vi "Launcher.vi"() -> ()   [LabVIEW 2019]
uses:
  <vilib>/ActorFramework/Message Enqueuer/Message Enqueuer.lvclass
  Status Actor/Status Actor.lvclass
  C:/Program Files/National Instruments/LabVIEW 2019/vi.lib/ActorFramework/Actor/Actor.lvclass
  Generador de funciones/Generador de funciones.lvclass
  <vilib>/ActorFramework/Message Enqueuer/Message Enqueuer.lvclass/Message Enqueuer.ctl
  <vilib>/ActorFramework/Message Enqueuer/Enqueue.vi
  <vilib>/ActorFramework/Stop Msg/Stop Msg.lvclass
  C:/Program Files/National Instruments/LabVIEW 2019/vi.lib/ActorFramework/Message/Message.lvclass
  <vilib>/ActorFramework/Message Priority Queue/Priority Enqueue.vi
  <vilib>/ActorFramework/Actor/Actor.lvclass
panel:
  in  "Exit":bool
  in  "Active Actors":u16(ring) items=["", "1"]
  in  "Stop Selected Actor":bool
  in  "Tipo de Actor":u16(ring) items=["Select an actor", "Status Actor", "Generador Actor"]
  in  "New Actor":bool
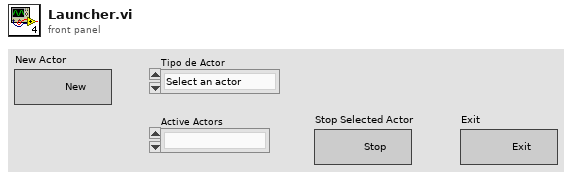
[diagram p1: front panel]
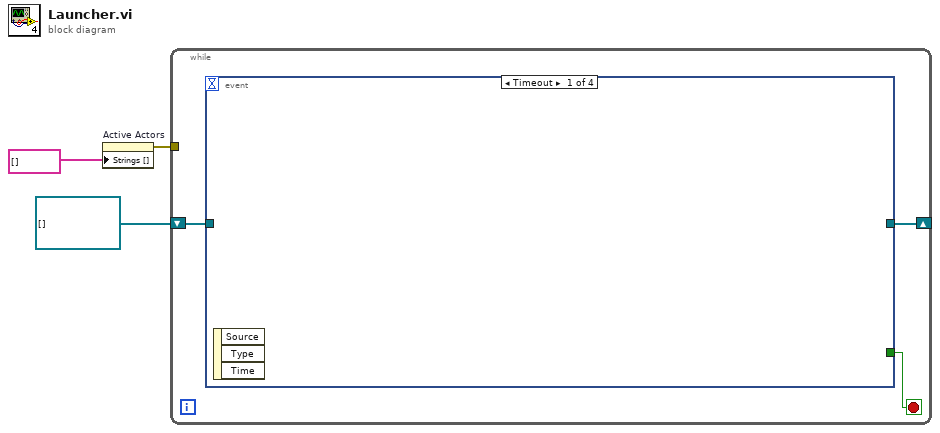
[diagram p0: block diagram]
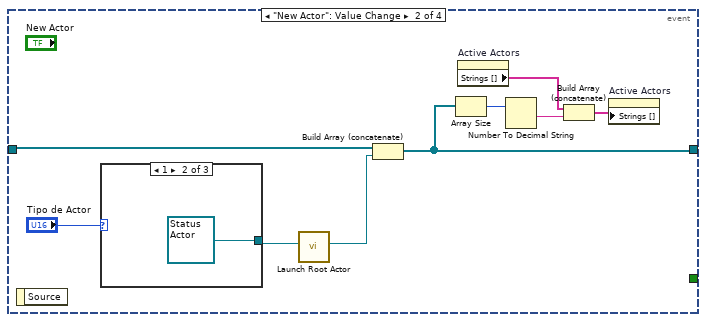
[diagram p2: hidden frame]
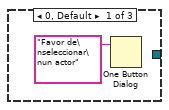
[diagram p3: hidden frame]
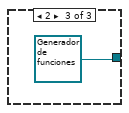
[diagram p4: hidden frame]
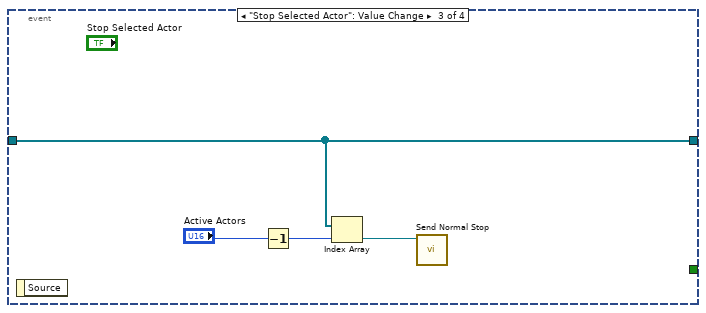
[diagram p5: hidden frame]
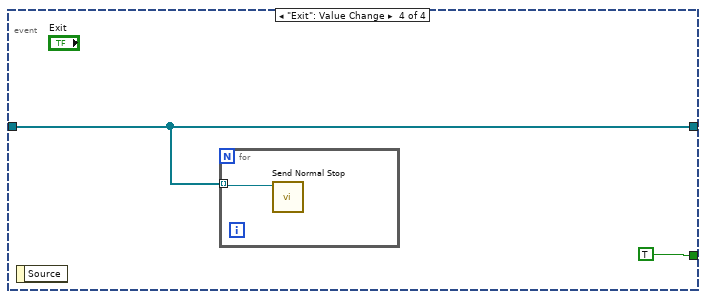
[diagram p6: hidden frame]
diagram:
  n1 = property on="Active Actors" class="Ring (strict)"("Strings []"=string[] []) -> (error out=w1:errorcluster)  [unwired: 2 in, 1 out]
  n2 = while {
    shift-right: [w5] -> _
    shift-left: refnum<class "Message Enqueuer.lvclass">[] [] ("Array") -> [w6]
    tunnel: w1 -> [_]
    stop <- w4 stop-if-true
    n3 = event shown="[0] Timeout" {
      selector: _ -> [_ _ _ _]
      dyn-events: _ -> [_ _ _ _]
      timeout: _ -> [_ _ _ _]
      tunnel: w6 -> [_ w12 w20 w23]
      tunnel: [_ w10 w20 w23] -> w5
      tunnel: [_ _ _ TRUE] -> w4
      event Timeout {
        n4 = event-data() -> ()  [unwired: 1 in, 3 out]
      }
      event "New Actor": Value Change {
        n5 = event-data() -> ()  [unwired: 1 in, 1 out]
        n6 = case shown="1" "Tipo de Actor" {
          tunnel: [_ refnum<class "Status Actor.lvclass"> refnum ("Status Actor.lvlib:Status Actor.lvclass") refnum<class "Generador de funciones.lvclass"> refnum ("Generador de funciones.lvlib:Generador de funciones.lvclass")] -> w13
          frame 0, Default {
            n7 = One Button Dialog(message="Favor de\nseleccionar\nun actor") -> ()  [unwired: 1 in, 1 out]
          }
          frame 1 {
          }
          frame 2 {
          }
        }
        n8 = call <vilib>:"Launch Root Actor.vi"("Actor"=w13) -> ("Actor's Enqueuer"=w11:refnum<class "Message Enqueuer.lvclass">)  [unwired: 9 in, 1 out]
        n9 = Build Array (concatenate)(w12, w11) -> (w10:refnum<class "Message Enqueuer.lvclass">[])
        n10 = Array Size(array=w10) -> (size(s)=w15:i32)
        n11 = property on="Active Actors" class="Ring (strict)"() -> ("Strings []"=w9:string[])  [unwired: 2 in, 2 out]
        n12 = Number To Decimal String(number=w15) -> (decimal integer string=w14:string)  [unwired: 1 in]
        n13 = Build Array (concatenate)(w9, w14) -> (w8:string[])
        n14 = property on="Active Actors" class="Ring (strict)"("Strings []"=w8) -> ()  [unwired: 2 in, 2 out]
      }
      event "Stop Selected Actor": Value Change {
        n15 = event-data() -> ()  [unwired: 1 in, 1 out]
        n16 = Decrement(x="Active Actors") -> (x-1=w22:u16)
        n17 = Index Array "Index Array"(array=w20, index=w22) -> (element=w19:refnum<class "Message Enqueuer.lvclass">)
        n18 = call <vilib>:"Send Normal Stop.vi"("Message Enqueuer"=w19) -> ()  [unwired: 10 in, 1 out]
      }
      event "Exit": Value Change {
        n19 = event-data() -> ()  [unwired: 1 in, 1 out]
        n20 = for {
          tunnel: w23 -> [w25] mode=indexing
          n21 = call <vilib>:"Send Normal Stop.vi"("Message Enqueuer"=w25) -> ()  [unwired: 10 in, 1 out]
        }
      }
    }
  }
